vi "Title Case.vi"(1 "String in":string) -> (0 "String out":string)   [LabVIEW 2015, in "ColorSelector.lvclass"]
doc: "This VI capitalizes the first character of each word.\n<b> </b> <b> </b>"
uses:
  ColorSelector.lvclass
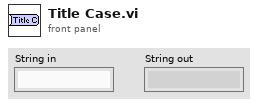
[diagram p1: front panel]
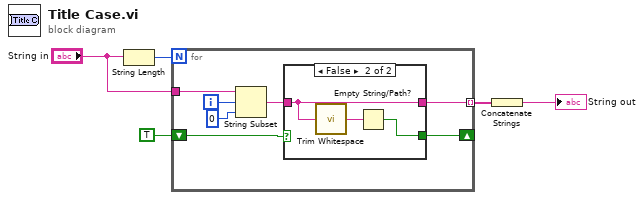
[diagram p0: block diagram]
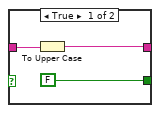
[diagram p2: hidden frame]
diagram:
  n1 = String Length(string="String in") -> (length=w4:i32)
  n2 = for {
    N: w4 -> [_]
    shift-right: [w11] -> _
    shift-left: TRUE -> [w12]
    tunnel: [w10] -> w2 mode=indexing
    tunnel: "String in" -> [w8]
    i -> [w7]
    n3 = String Subset(string=w8, offset (0)=w7, length (rest)=0 ("length (rest)")) -> (substring=w9:string)
    n4 = case shown="False" w12 {
      tunnel: w9 -> [w15 w18]
      tunnel: [w14 w18] -> w10
      tunnel: [FALSE w16] -> w11
      frame True {
        n5 = To Upper Case(1:w15) -> (0:w14:string)
      }
      frame False {
        n6 = call <vilib>:"Trim Whitespace.vi"("string"=w18) -> ("trimmed string"=w17:string)  [unwired: 1 in]
        n7 = Empty String/Path?(string/path=w17) -> (empty?=w16:bool)
      }
    }
  }
  n8 = Concatenate Strings(w2) -> (→"String out":string)
